vi "Redukuj opisy nieaktywne.vi"(7 "Aktywne in":bool[](array[boolean]), 8 "error in (no error)":errorcluster, 10 "Opisy in":string[](array[string])) -> (0 "error out":errorcluster, 2 "Opisy out":string[](array[string]))   [LabVIEW 2014]
doc: "Redukuje opisy tylko do aktywnych kana丑w"
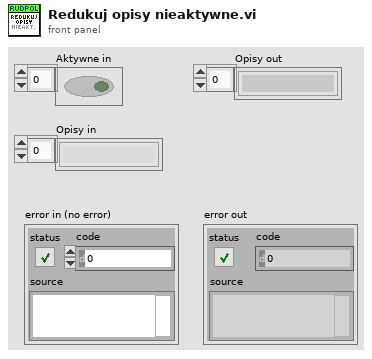
[diagram p1: front panel]
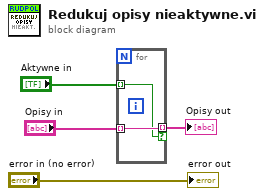
[diagram p0: block diagram]
diagram:
  n1 = for {
    tunnel: "Aktywne in" -> [w5] mode=indexing
    tunnel: "Opisy in" -> [w6] mode=indexing
    tunnel: [w6] -> w4 mode=indexing if=w5
  }
  "Opisy out" <- w4
  "error out" <- "error in (no error)"
